vi "Task.vi"(8 "error in (no error)":cluster{"状态":bool, "代码":i32, "源":string} caption="错误输入（无错误）", 10 "数据":i32, 11 "Beta输入":refnum<class "Beta.lvclass">) -> (0 "error out":cluster{"状态":bool, "代码":i32, "源":string} caption="错误输出", 3 "Beta输出":refnum<class "Beta.lvclass">)   [LabVIEW 2013, in "Beta操作者.lvlib" / "Beta.lvclass"]
uses:
  Beta.lvclass
  <vilib>/ActorFramework/Actor/Actor.lvclass
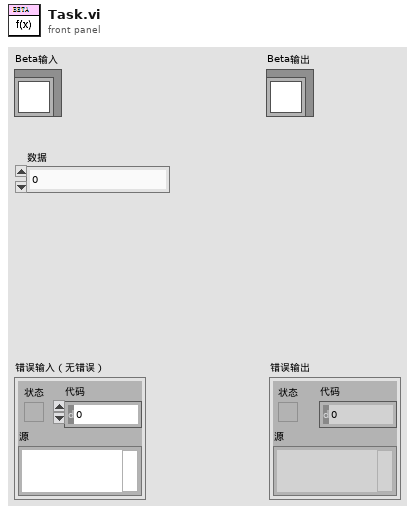
[diagram p1: front panel]
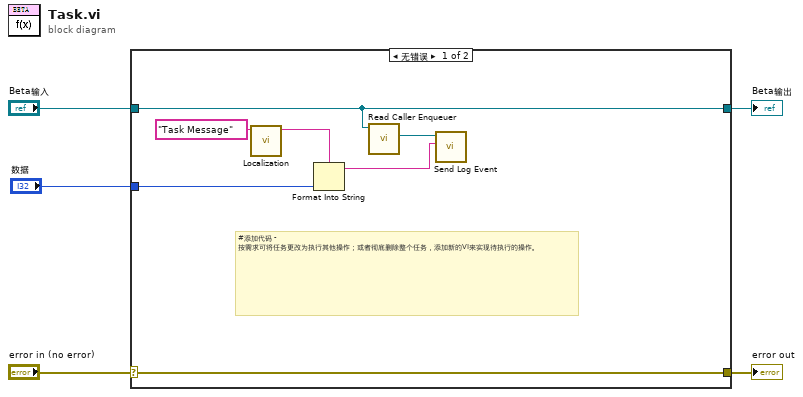
[diagram p0: block diagram]
diagram:
  n1 = case shown="无错误" "error in (no error)" {
    selector: "error in (no error)" -> [w12 w14]
    tunnel: [w12 w14] -> w4
    tunnel: [w11 w13] -> w2
    tunnel: "Beta输入" -> [w11 w13]
    tunnel: "数据" -> [w7 _]
    frame No Error {
      # "#添加代码 - 按需求可将任务更改为执行其他操作；或者彻底删除整个任务，添加新的VI来实现待执行的操作。"
      n2 = call "Localization.vi"("未本地化"="Task Message" ("Unlocalized")) -> ("本地化"=w8:string)  [unwired: 10 in]
      n3 = Format Into String(format string=w8, w7) -> (resulting string=w6:string)  [unwired: 2 in, 1 out]
      n4 = call <vilib>:"Read Caller Enqueuer.vi"("Actor"=w11) -> ("Caller Enqueuer"=w10:refnum<class "Message Enqueuer.lvclass">)  [unwired: 10 in]
      n5 = call "Send Log Event.vi"("事件文本"=w6, "消息待入队列"=w10) -> ()  [unwired: 9 in, 1 out]
    }
    frame Error {
    }
  }
  "error out" <- w4
  "Beta输出" <- w2
